vi "Import Raw Pictures.vi"(0 "Display State In":T2, 5 "Pictures Data":T1[](array[typedef]), 9 "Container State":T4, 11 "error in (no error)":errorcluster) -> (4 "Display State Out":T2, 15 "error out":errorcluster)   [LabVIEW 2016]
uses:
  <vilib>/_xctls/Container State.ctl
  <vilib>/_xctls/XControlSupport.lvlib
  <vilib>/Utility/miscctls.llb/LVBoundsTypeDef.ctl
  HorizontalList_State.ctl
  HorizontalList.xctl
  <vilib>/picture/picture.llb/imagedata.ctl
panel:
  out "Array":picture[](array[picture])
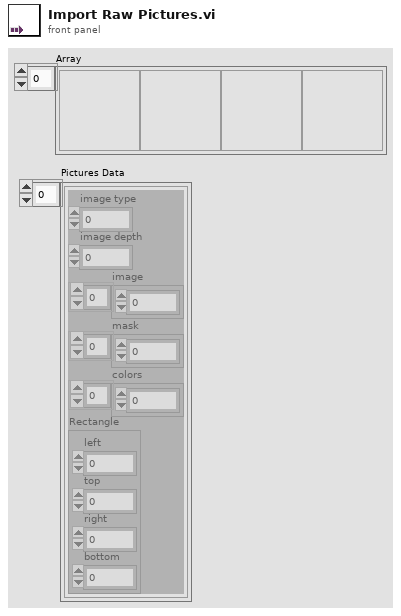
[diagram p1: front panel]
types:
  T1 = typedef "imagedata.ctl" = cluster{"image type":i32, "image depth":i32, "image":u8[], "mask":u8[], "colors":u32[], "Rectangle":cluster{"left":i16, "top":i16, "right":i16, "bottom":i16}}
  T2 = typedef "HorizontalList.xctl/HorizontalList_State.ctl" = cluster{"Persistent":cluster{"Elements":string[], "PicElements":picture[], "Limits":i32[], "Selection":picture[], "Selection Color":u32, "Highlight":picture[], "Highlight Val":i32, "Highlight Color":u32}, "Draw Area Size":T3, "List Ref":refnum<vi>, "Visible":u8}
  T3 = typedef "LVBoundsTypeDef.ctl" = cluster{"Width":u32, "Height":u32}
  T4 = typedef "XControlSupport.lvlib/Container State.ctl" = cluster{"Indicator?":bool, "Run Mode?":bool, " Refnum":refnum<vi>}
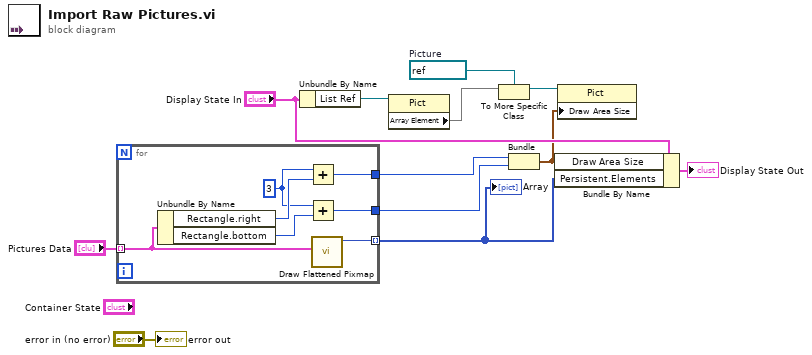
[diagram p0: block diagram]
diagram:
  w6 = refnum<vi> refnum  # Picture
  n1 = for {
    tunnel: [w19] -> w11 mode=indexing
    tunnel: "Pictures Data" -> [w18] mode=indexing
    tunnel: [w14] -> w4
    tunnel: [w13] -> w3
    w15 = i16 3 ("x")
    n2 = Unbundle By Name(w18) -> ("Rectangle.right"=w16:i16, "Rectangle.bottom"=w17:i16)
    n3 = Add(x=w15, y=w16) -> (x+y=w14:i16)
    n4 = Add(x=w15, y=w17) -> (x+y=w13:i16)
    n5 = call <vilib>:"Draw Flattened Pixmap.vi"("image data"=w18) -> ("new picture"=w19:picture)  [unwired: 8 in]
  }
  "Array" <- w11
  n6 = Unbundle By Name("Display State In") -> ("List Ref"=w8:refnum<vi>)
  n7 = property class="Pict"(reference=w8) -> ("Array Element"=w7)  [unwired: 1 in, 2 out]
  n8 = To More Specific Class(target class=w6, reference=w7) -> (specific class reference=w5:refnum<vi>)  [unwired: 1 in, 1 out]
  n9 = Bundle(w4, w3) -> (w2:cluster{i16, i16})  [unwired: 1 in]
  n10 = Bundle By Name(cluster="Display State In", "Draw Area Size"=w2, "Persistent.Elements"=w11) -> (→"Display State Out":T2)
  n11 = property class="Pict"(reference=w5, "Draw Area Size"=w2) -> ()  [unwired: 1 in, 2 out]
  "error out" <- "error in (no error)"
